vi "KV_VolHead_ReadVol.vi"(10 "地址":u8=1 min=1 max=10 step=1, 11 "MyIndex":u8) -> (3 "Value":dbl)   [LabVIEW 2015]
uses:
  <vilib>/Instr/_visa.llb/VISA Configure Serial Port (Instr).vi
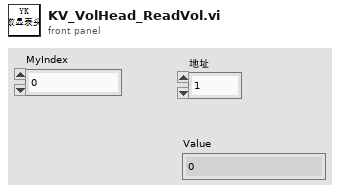
[diagram p1: front panel]
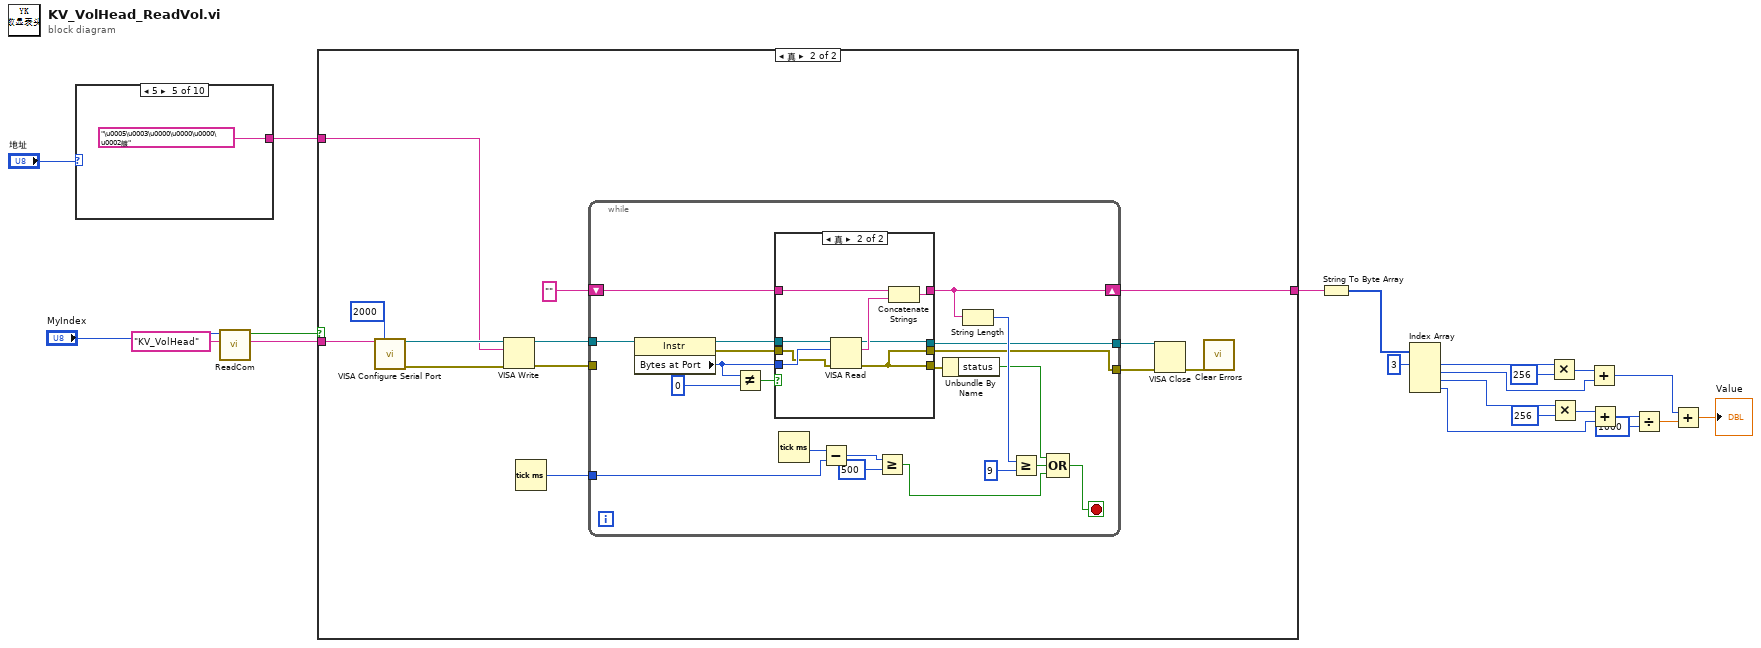
[diagram p0: block diagram]
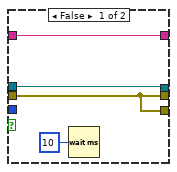
[diagram p3: hidden frame]
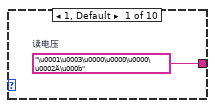
[diagram p4: hidden frame]
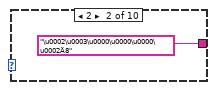
[diagram p5: hidden frame]
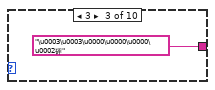
[diagram p6: hidden frame]
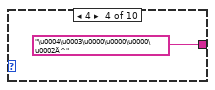
[diagram p7: hidden frame]
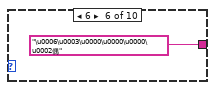
[diagram p8: hidden frame]
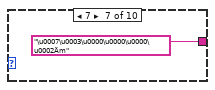
[diagram p9: hidden frame]
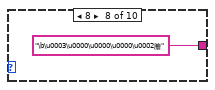
[diagram p10: hidden frame]
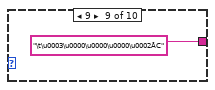
[diagram p11: hidden frame]
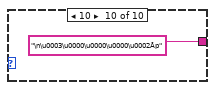
[diagram p12: hidden frame]
diagram:
  n1 = case shown="5" "地址" {
    tunnel: [w23 "\u0002\u0003\u0000\u0000\u0000\u0002Ä8" ("写入缓冲区") "\u0003\u0003\u0000\u0000\u0000\u0002砰" ("写入缓冲区") "\u0004\u0003\u0000\u0000\u0000\u0002Ä^" ("写入缓冲区") "\u0005\u0003\u0000\u0000\u0000\u0002艔" ("写入缓冲区") "\u0006\u0003\u0000\u0000\u0000\u0002偶" ("写入缓冲区") "\u0007\u0003\u0000\u0000\u0000\u0002Äm" ("写入缓冲区") "\b\u0003\u0000\u0000\u0000\u0002膾" ("写入缓冲区") "\t\u0003\u0000\u0000\u0000\u0002ÅC" ("写入缓冲区") "\n\u0003\u0000\u0000\u0000\u0002Åp" ("写入缓冲区")] -> w22
    frame 1, Default {
      w23 = "\u0001\u0003\u0000\u0000\u0000\u0002Ä\u000b"  # 读电压
    }
    frame 2 {
    }
    frame 3 {
    }
    frame 4 {
    }
    frame 5 {
    }
    frame 6 {
    }
    frame 7 {
    }
    frame 8 {
    }
    frame 9 {
    }
    frame 10 {
    }
  }
  n2 = call "ReadCom.vi"("仪器名称"="KV_VolHead", "MyIndex"="MyIndex") -> ("COM"=w2:string, "OK?"=w1:bool)  [unwired: 7 in, 1 out]
  n3 = case shown="真" w1 {
    tunnel: w22 -> [_ w43]
    tunnel: [_ w38] -> w5
    tunnel: w2 -> [_ w36]
    frame False {
    }
    frame True {
      n4 = call-poly "VISA Configure Serial Port"("VISA resource name"=w36, "timeout (10sec)"=u32 2000) -> ("VISA resource name out"=w45:refnum<visa-resource-name>, "error out"=w44:errorcluster)  [unwired: 12 in]
      n5 = VISA Write(VISA resource name=w45, write buffer=w43, error in (no error)=w44) -> (VISA resource name out=w41:refnum<visa-resource-name>, error out=w42:errorcluster)  [unwired: 1 out]
      n6 = Tick Count (ms)() -> (millisecond timer value=w39:u32)
      n7 = while {
        tunnel: w42 -> [_]
        tunnel: w41 -> [w66]
        shift-right: [w59] -> w38
        shift-left: "" -> [w60]
        tunnel: w39 -> [w51]
        tunnel: [w47] -> w35
        tunnel: [w46] -> w34
        stop <- w55 stop-if-true
        n8 = property class="Instr"(reference=w66) -> (reference out=w63:refnum<visa-resource-name>, error out=w61:errorcluster, "Bytes at Port"=w62:u32)  [unwired: 1 in]
        n9 = Not Equal?(x=w62, y=u32 0) -> (x != y?=w64:bool)
        n10 = case shown="真" w64 {
          tunnel: w63 -> [w68 w78]
          tunnel: w62 -> [_ w77]
          tunnel: w61 -> [w67 w76]
          tunnel: w60 -> [w69 w75]
          tunnel: [w69 w73] -> w59
          tunnel: [w67 w71] -> w54
          tunnel: [w68 w72] -> w47
          tunnel: [w67 w71] -> w46
          frame False {
            n11 = Wait (ms)(milliseconds to wait=u32 10 ("等待时间（毫秒）")) -> ()  [unwired: 1 out]
          }
          frame True {
            n12 = VISA Read(VISA resource name=w78, byte count=w77, error in (no error)=w76) -> (VISA resource name out=w72:refnum<visa-resource-name>, read buffer=w74:string, error out=w71:errorcluster)  [unwired: 1 out]
            n13 = Concatenate Strings(w75, w74) -> (w73:string)
          }
        }
        n14 = Tick Count (ms)() -> (millisecond timer value=w52:u32)
        n15 = Subtract(x=w52, y=w51) -> (x-y=w50:u32)
        n16 = Greater Or Equal?(x=w50, y=u32 500) -> (x >= y?=w48:bool)
        n17 = Unbundle By Name(w54) -> ("status"=w53:bool)
        n18 = String Length(string=w59) -> (length=w58:i32)
        n19 = Greater Or Equal?(x=w58, y=9) -> (x >= y?=w57:bool)
        n20 = Compound Arithmetic op=OR ("复合运算")(w53, w57, w48) -> (w55:bool)
      }
      n21 = VISA Close(VISA resource name=w35, error in (no error)=w34) -> (error out=w33:errorcluster)
      n22 = call <vilib>:"Clear Errors.vi"("error in (no error)"=w33) -> ()  [unwired: 5 in, 2 out]
    }
  }
  n23 = String To Byte Array(string=w5) -> (unsigned byte array=w7:u8[])
  n24 = Index Array(array=w7, index #1=3 ("索引")) -> (element #1=w20:u8, element #2=w17:u8, element #3=w14:u8, element #4=w13:u8)  [unwired: 3 in]
  n25 = Multiply(x=w20, y=i16 256) -> (x*y=w18:i16)
  n26 = Multiply(x=w14, y=i16 256) -> (x*y=w16:i16)
  n27 = Add(x=w18, y=w17) -> (x+y=w9:i16)
  n28 = Add(x=w16, y=w13) -> (x+y=w12:i16)
  n29 = Divide(x=w12, y=i16 1000) -> (x/y=w10:dbl)
  n30 = Add(x=w9, y=w10) -> (x+y=→"Value":dbl)
